vi "PCO_ControlCommandCall.vi"(0 "ph":u64, 5 "buf_in":u8[](array[numeric]), 11 "error in (no error)":errorcluster {"code" format="%x"}) -> (4 "ph out":u64, 6 "ErrorMessage":i32 format="%x", 10 "buf_out":u8[](array[numeric]), 15 "error out":errorcluster {"code" format="%x"})   [LabVIEW 2019, in "SDK.lvlib" / "GeneralCameraControl.lvlib"]
doc: "<b>Description:</b>\nThis function issues a low level command to the camera. This call is part of most of the other calls. Normally calling this function is not needed. It can be used to cover those camera commands, which are not implemented in regular SDK functions.\n\n<b>Supported camera type:</b>\nAll cameras\n\n<b>Descriptor dependency:</b>\nNone"
uses:
  GeneralCameraControl.lvlib
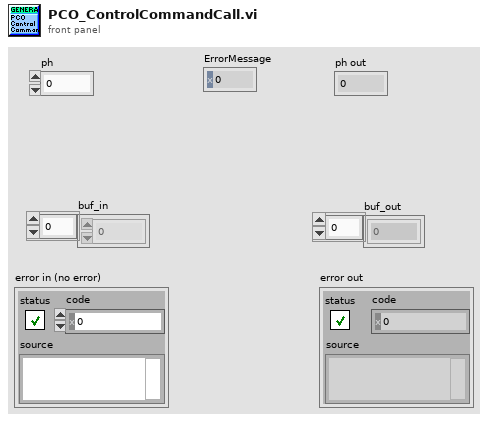
[diagram p1: front panel]
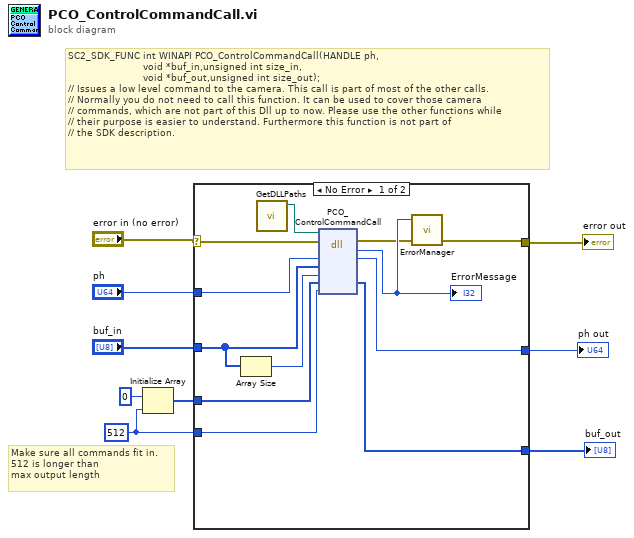
[diagram p0: block diagram]
diagram:
  w1 = u32 512
  # "Make sure all commands fit in.\n512 is longer than \nmax output length"
  # "SC2_SDK_FUNC int WINAPI PCO_ControlCommandCall(HANDLE ph,\n                         void *buf_in,unsigned int size_in,\n                         void *buf_out,unsigned int size_out);\n// Issues a low level command to the camera. This call is part of most of the other calls.\n// Normally you do not need to call this function. It can be used to cover those camera\n// commands, which are not part of this Dll up to now. Please use the other functions while\n// their purpose is easier to understand. Furthermore this function is not part of\n// the SDK description."
  n1 = Initialize Array(u8 0 ("element"), w1) -> (w4:u8[])
  n2 = case shown="No Error" "error in (no error)" {
    selector: "error in (no error)" -> [w15 w22]
    tunnel: "ph" -> [w21 w23]
    tunnel: [w20 w23] -> w8
    tunnel: [w19 w22] -> w7
    tunnel: [w17 w24] -> w6
    tunnel: w1 -> [w16 _]
    tunnel: w4 -> [w13 w24]
    tunnel: "buf_in" -> [w12 _]
    frame No Error {
      n3 = Array Size(array=w12) -> (size(s)=w11:i32)
      n4 = call "GetDLLPaths.vi"() -> ("SC2_Cam_Path"=w10:path)  [unwired: 9 in, 2 out]
      n5 = dll-call lib="?" fn="PCO_ControlCommandCall"(path in=w10, error in=w15, "ph"=w21, "buf_in"=w12, "size_in"=w11, "buf_out"=w13, "size_out"=w16) -> (error out=w14:errorcluster, "return type"=w18:i32, "ph"=w20:u64, "buf_out"=w17:u8[])  [unwired: 4 in, 1 out]
      "ErrorMessage" <- w18
      n6 = call "ErrorManager.vi"("error in (no error)"=w14, "error code"=w18) -> ("error out"=w19:errorcluster)  [unwired: 3 in]
    }
    frame Error {
    }
  }
  "ph out" <- w8
  "error out" <- w7
  "buf_out" <- w6
